vi "compare.vi"(1 "Value 2":dbl, 2 "Value 1":dbl, 3 "Tolerance":dbl) -> (0 "Comparison":bool)   [LabVIEW 2019]
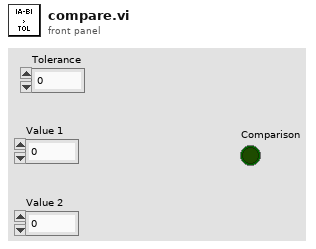
[diagram p1: front panel]
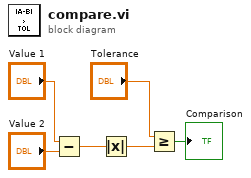
[diagram p0: block diagram]
diagram:
  n1 = Subtract(x="Value 1", y="Value 2") -> (x-y=w4:dbl)
  n2 = Absolute Value(x=w4) -> (abs(x)=w1:dbl)
  n3 = Greater Or Equal?(x="Tolerance", y=w1) -> (x >= y?=→"Comparison":bool)
